vi "Create Instrument Addon.vi"() -> ()   [LabVIEW 2018, in "Instrument Addon Scripting API.lvlib"]
uses:
  Instrument Addon Scripting API.lvlib
  NationalInstruments.VeriStand.SystemDefinitionAPI
  Addon/Addon Shared/SubVIs/Constants.vi
  Addon/Addon Shared/Instrument Addon Shared.lvlib
  <vilib>/NI Veristand/Custom Device Tools/Custom Device Utility Library/Custom Device Utility Library.lvlib
  Addon/Support Libraries/Protocols.lvlibp/Protocol Parent/Protocol Parent.lvclass
panel:
  in  "PCL Decimation":i32
  out "error out":errorcluster={"status"=TRUE, "code"=7, "source"="Open VI Reference in Custom Device API.lvlib:NI VeriStand - Find next valid Label.vi->Instrument Addon Scripting API.lvlib:Create Instrument Addon.vi<APPEND>\nVI Path: <b>C:\\Program Files (x86)\\National Instruments\\LabVIEW 2018\\vi.lib\\NI VeriStand\\Custom Device Offline API\\NI VeriStand - Find next valid Label.vi</b>"}
  in  "error in (no error) 3":errorcluster
  out "Target Out":refnum<k24>
  in  "error in (no error)":errorcluster
  in  "Target In":refnum<k24>
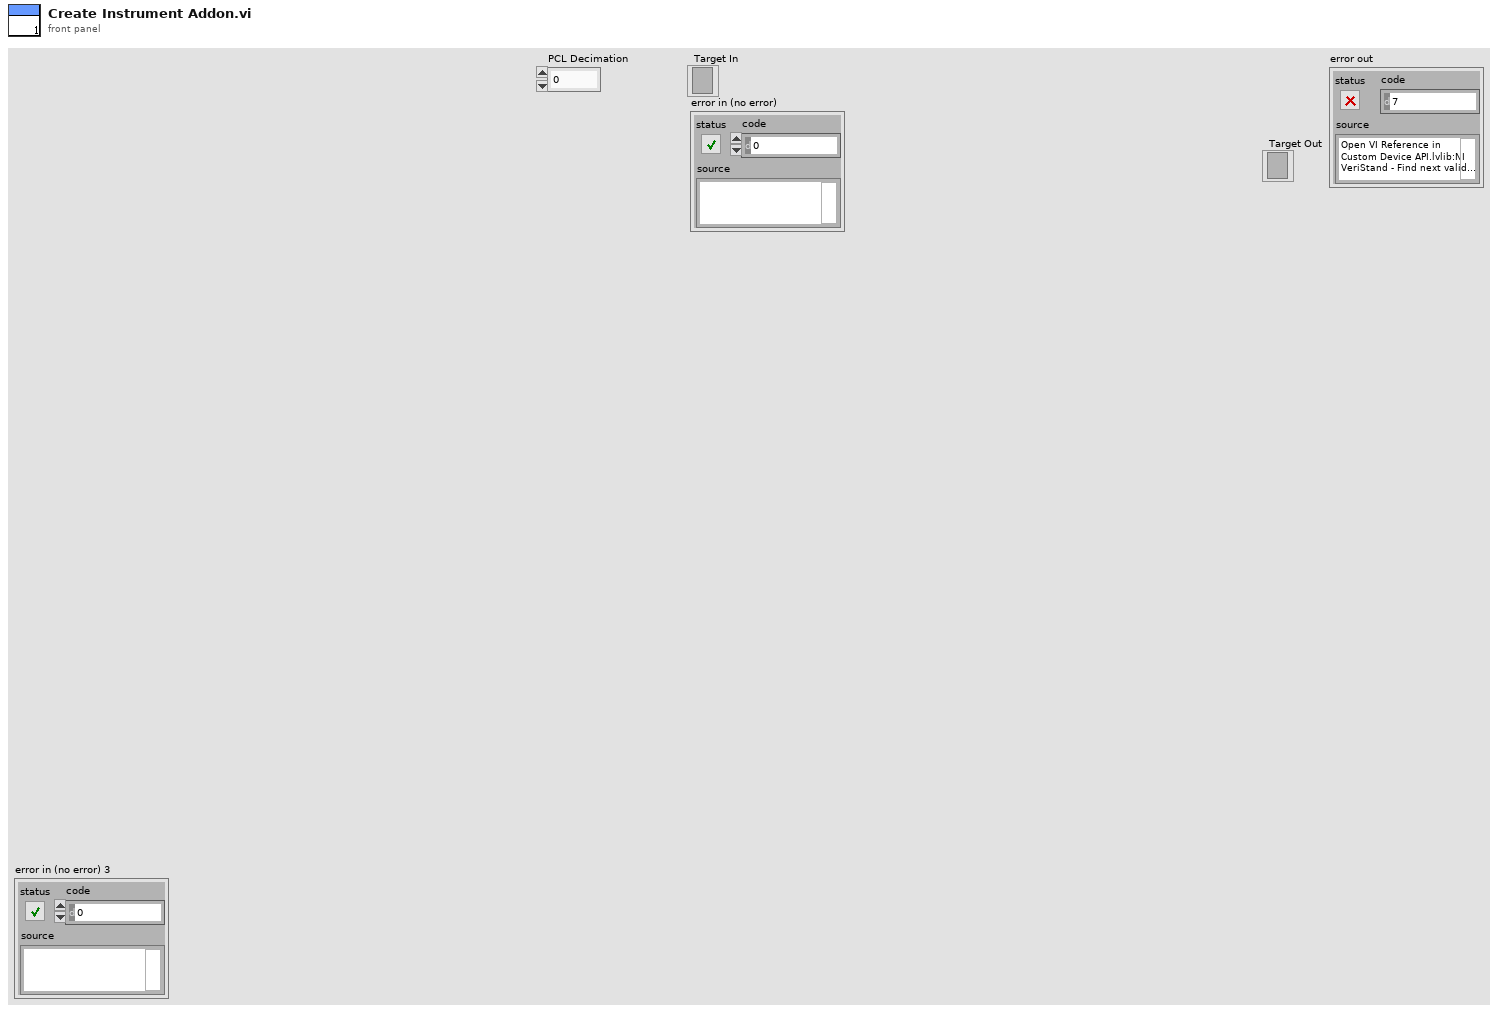
[diagram p1: front panel]
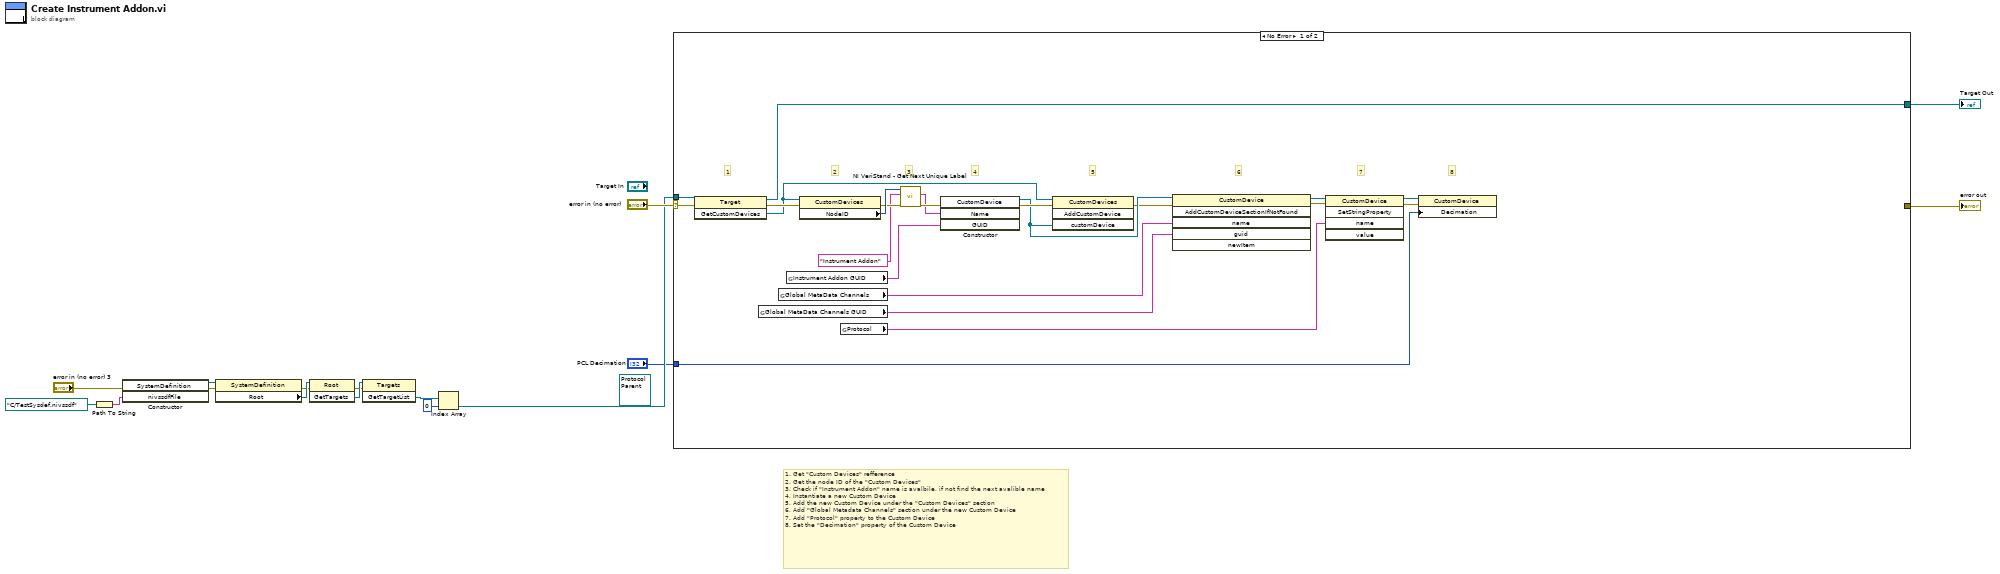
[diagram p0: block diagram]
diagram:
  (unwired) refnum<class "Protocol Parent.lvclass"> refnum ("Protocols.lvlibp:Protocol Parent.lvclass")
  # "1. Get \"Custom Devices\" refference\n2. Get the node ID of the \"Custom Devices\" \n3. Check if \"Instrument Addon\" name is avalbile, if not find the next avalible name\n4. Instantiate a new Custom Device\n5. Add the new Custom Device under the \"Custom Devices\" section\n6. Add \"Global Metadata Channels\" section under the new Custom Device\n7. Add \"Protocol\" property to the Custom Device\n8. Set the \"Decimation\" property of the Custom Device"
  n1 = Path To String(path=path "C:/TestSysdef.nivssdf") -> (string=w11:string)
  n2 = constructor class="SystemDefinition"(error in="error in (no error) 3", "nivssdfFile"=w11) -> (reference out=w3:refnum<k24>, error out=w13:errorcluster)  [unwired: 2 in, 2 out]
  n3 = property class="SystemDefinition"(reference=w3, error in=w13) -> (error out=w7:errorcluster, "Root"=w8:refnum<k24>)  [unwired: 1 out]
  n4 = invoke class="Root" method="GetTargets"(reference=w8, error in=w7) -> (error out=w9:errorcluster, "GetTargets"=w10:refnum<k24>)  [unwired: 1 in, 1 out]
  n5 = invoke class="Targets" method="GetTargetList"(reference=w10, error in=w9) -> ("GetTargetList"=w6:refnum<k24>[])  [unwired: 1 in, 2 out]
  n6 = Index Array(array=w6, index=0) -> (element=w2:refnum<k24>)
  n7 = case shown="No Error" "error in (no error)" {
    selector: "error in (no error)" -> [w37 w39]
    tunnel: w2 -> [w38 w40]
    tunnel: [w36 w40] -> w15
    tunnel: [_ w39] -> w4
    tunnel: "PCL Decimation" -> [w22 _]
    frame No Error {
      # "8"
      # "7"
      # "6"
      # "5"
      # "4"
      # "3"
      # "2"
      # "1"
      n8 = invoke class="Target" method="GetCustomDevices"(reference=w38, error in=w37) -> (reference out=w36:refnum<k24>, error out=w33:errorcluster, "GetCustomDevices"=w27:refnum<k24>)  [unwired: 1 in]
      n9 = global read "Constants.vi" "Global MetaData Channels GUID"() -> (w23:string)
      n10 = global read "Constants.vi" "Global MetaData Channels"() -> (w24:string)
      n11 = global read "Constants.vi" "Instrument Addon GUID"() -> (w35:string)
      n12 = property class="CustomDevices"(reference=w27, error in=w33) -> (error out=w31:errorcluster, "NodeID"=w32:u64)  [unwired: 1 out]
      n13 = global read "Constants.vi" "Protocol"() -> (w21:string)
      n14 = call <vilib>:"NI VeriStand - Get Next Unique Label.vi"("error in (no error)"=w31, "Label"="Instrument Addon", "Parent Ref in"=w32) -> ("error out"=w29:errorcluster, "Label out"=w28:string)  [unwired: 5 in, 2 out]
      n15 = constructor class="CustomDevice"(error in=w29, "Name"=w28, "GUID"=w35) -> (reference out=w26:refnum<k24>, error out=w34:errorcluster)  [unwired: 2 in, 3 out]
      n16 = invoke class="CustomDevices" method="AddCustomDevice"(reference=w27, error in=w34, "customDevice"=w26) -> (error out=w25:errorcluster)  [unwired: 1 in, 3 out]
      n17 = invoke class="CustomDevice" method="AddCustomDeviceSectionIfNotFound"(reference=w26, error in=w25, "name"=w24, "guid"=w23) -> (reference out=w19:refnum<k24>, error out=w20:errorcluster)  [unwired: 2 in, 4 out]
      n18 = invoke class="CustomDevice" method="SetStringProperty"(reference=w19, error in=w20, "name"=w21) -> (reference out=w17:refnum<k24>, error out=w18:errorcluster)  [unwired: 2 in, 3 out]
      n19 = property class="CustomDevice"(reference=w17, error in=w18, "Decimation"=w22) -> ()  [unwired: 2 out]
    }
    frame Error {
    }
  }
  "Target Out" <- w15
  "error out" <- w4
